vi "New Entity.vi"(7 "Entity Type":refnum<class "Entity.lvclass">, 8 "error in (no error)":errorcluster, 11 "Entity Manager in":refnum<class "Entity Manager.lvclass">) -> (0 "error out":errorcluster, 2 "Entity":refnum<class "Entity.lvclass">, 3 "Entity Manager out":refnum<class "Entity Manager.lvclass">)   [LabVIEW 2020, in "Conditu2.lvlib" / "Entity Manager.lvclass"]
uses:
  Entity Manager.lvclass
  Entity/Entity.lvclass
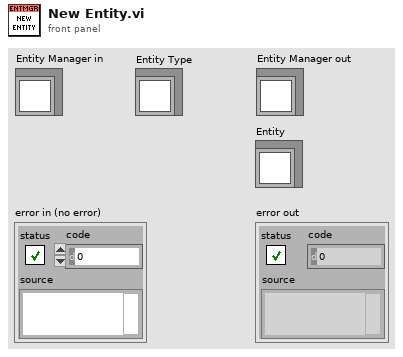
[diagram p1: front panel]
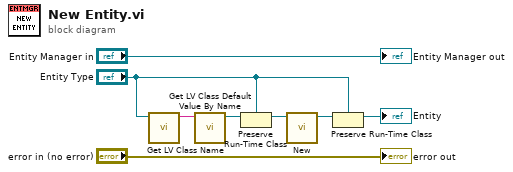
[diagram p0: block diagram]
diagram:
  n1 = call <vilib>:"Get LV Class Name.vi"("object"="Entity Type") -> ("class name"=w4:string)  [unwired: 9 in, 1 out]
  n2 = call <vilib>:"Get LV Class Default Value By Name.vi"("class name"=w4) -> ("object"=w3:refnum<class>)  [unwired: 9 in, 1 out]
  n3 = Preserve Run-Time Class(object in=w3, 2:"Entity Type") -> (object out=w1:refnum<class "Entity.lvclass">)  [unwired: 1 in, 1 out]
  n4 = call "New.vi"("Entity in"=w1) -> ("Entity out"=w6:refnum<class "Entity.lvclass">)  [unwired: 10 in]
  n5 = Preserve Run-Time Class(object in=w6, 2:"Entity Type") -> (object out=→"Entity":refnum<class "Entity.lvclass">)  [unwired: 1 in, 1 out]
  "error out" <- "error in (no error)"
  "Entity Manager out" <- "Entity Manager in"
